vi "read serial number (module EEPROM).vi"(8 "error in":errorcluster, 11 "Refnum in":refnum<k20>) -> (0 "error out":errorcluster, 1 "Serial Number":u32 format="%x", 2 "Serial Number String":string, 3 "Refnum out":refnum<k20>)   [LabVIEW 2016, in "SMI.lvlib" / "C Series Module.lvclass"]
uses:
  C Series Module.lvclass
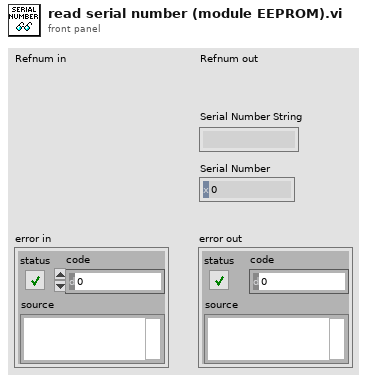
[diagram p1: front panel]
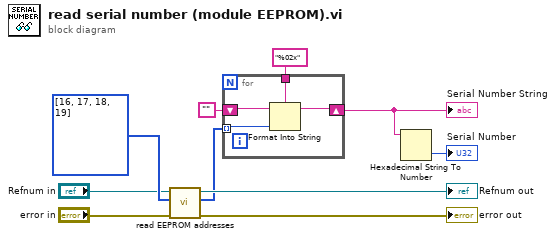
[diagram p0: block diagram]
diagram:
  n1 = call "read EEPROM addresses.vi"("error in (no error)"="error in", "Addresses"=u16[] [16, 17, 18, 19], "Refnum in"="Refnum in") -> ("error out"=→"error out":errorcluster, "Data"=w4:u8[], "Refnum out"=→"Refnum out":refnum<k20>)  [unwired: 6 in]
  n2 = for {
    tunnel: "%02x" ("format string") -> [w14]
    tunnel: w4 -> [w13] mode=indexing
    shift-right: [w12] -> w2
    shift-left: "" -> [w11]
    n3 = Format Into String(format string=w14, initial string=w11, w13) -> (resulting string=w12:string)  [unwired: 1 in, 1 out]
  }
  "Serial Number String" <- w2
  n4 = Hexadecimal String To Number(string=w2) -> (number=→"Serial Number":u32)  [unwired: 2 in, 1 out]
